vi "Selection Handle Mouse Down.vi"(7 "Shift?":bool, 8 "error in (no error)":errorcluster, 9 "Mouse Button":u16, 10 "Mouse Coords":T1, 11 "Listbox or Tree":refnum<vi>) -> (0 "error out":errorcluster, 3 "Discard?":bool)   [LabVIEW 2020, in "UI_ItemSelect.lvlib"]
uses:
  UI_ItemSelect.lvlib
  <vilib>/Utility/miscctls.llb/LVPoint32TypeDef.ctl
  SubVIs/item select mouse down data.ctl
  SubVIs/item select action.ctl
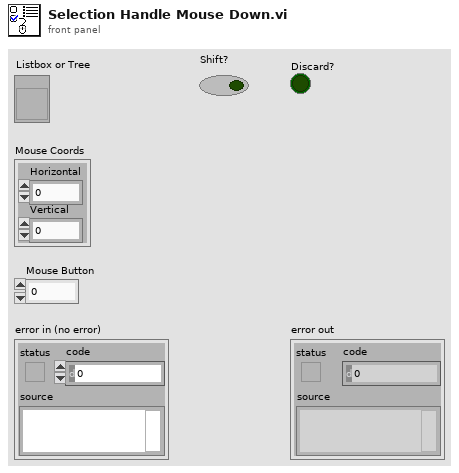
[diagram p1: front panel]
types:
  T1 = typedef "LVPoint32TypeDef.ctl" = cluster{"Horizontal":i32, "Vertical":i32}
  T2 = typedef "UI_ItemSelect.lvlib/item select action.ctl" = enum16{"init", "read", "write states", "write locks", "mouse down", "delete", "select all", "select none", "invert selection"}
  T3 = typedef "UI_ItemSelect.lvlib/item select mouse down data.ctl" = cluster{"Shift":bool, "Selected Row":i32}
  T4 = typedef "LVRowAndColumnTypeDef.ctl" = cluster{"Row":i32, "Column":i32}
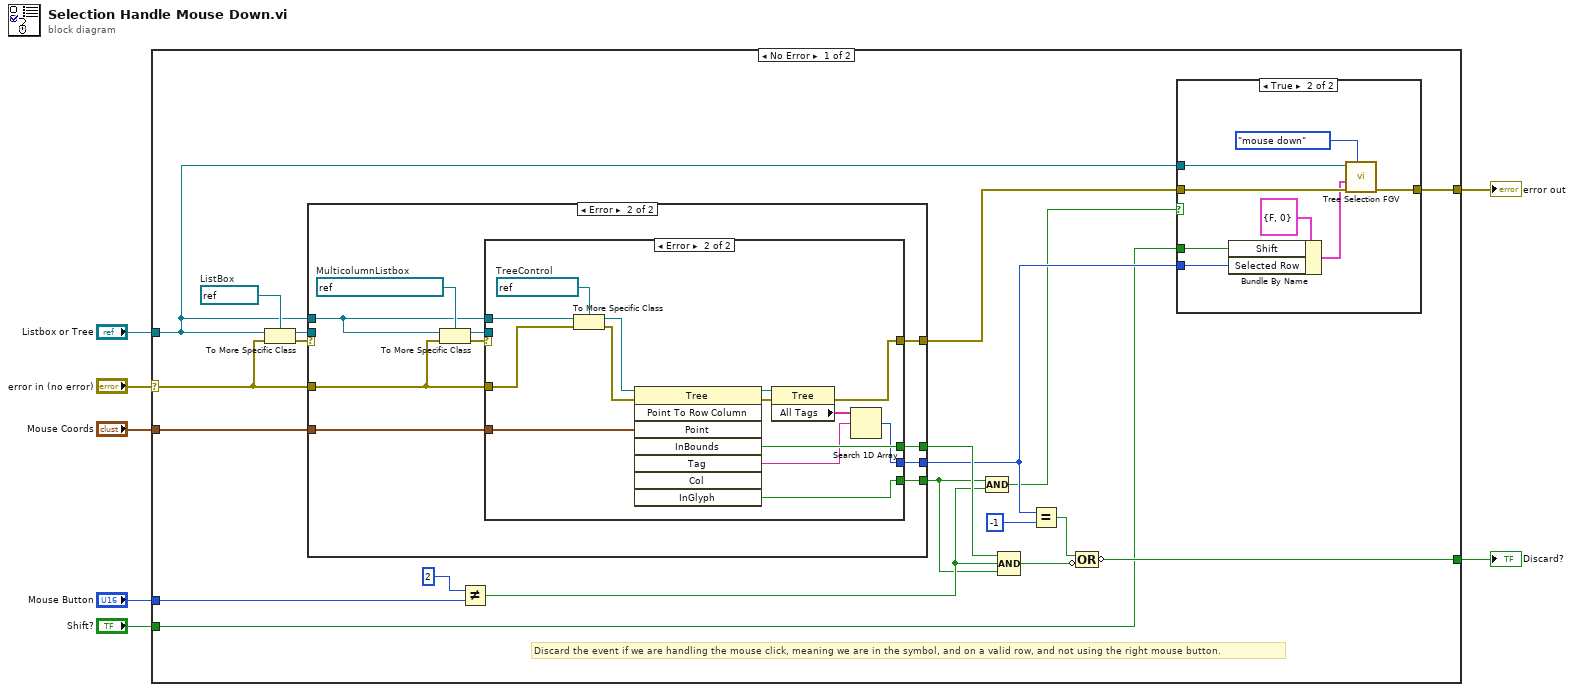
[diagram p0: block diagram]
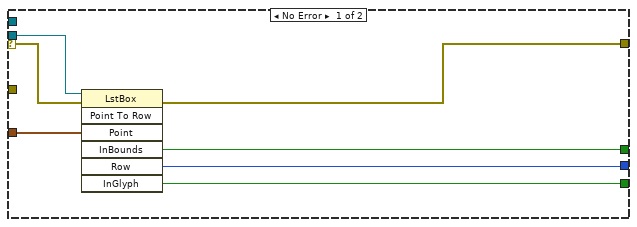
[diagram p2: hidden frame]
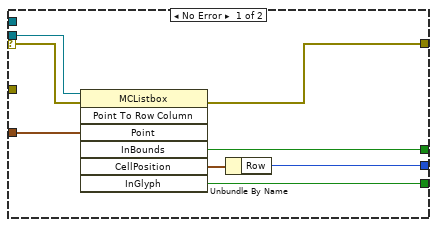
[diagram p3: hidden frame]
diagram:
  n1 = case shown="No Error" "error in (no error)" {
    selector: "error in (no error)" -> [w24 w76]
    tunnel: [w12 w76] -> w7
    tunnel: "Listbox or Tree" -> [w9 _]
    tunnel: "Mouse Coords" -> [w23 _]
    tunnel: "Mouse Button" -> [w22 _]
    tunnel: [w11 _] -> w2
    tunnel: "Shift?" -> [w10 _]
    frame No Error {
      w25 = refnum<vi> refnum  # ListBox
      # "Discard the event if we are handling the mouse click, meaning we are in the symbol, and on a valid row, and not using the right mouse button."
      n2 = To More Specific Class(target class=w25, reference=w9, error in=w24) -> (specific class reference=w27:refnum<vi>, error out=w26:errorcluster)
      n3 = case shown="Error" w26 {
        selector: w26 -> [w33 _]
        tunnel: w27 -> [w34 _]
        tunnel: w24 -> [_ w35]
        tunnel: [w32 w42] -> w15
        tunnel: w23 -> [w31 w41]
        tunnel: [w30 w39] -> w8
        tunnel: [w29 w40] -> w14
        tunnel: [w28 w38] -> w20
        tunnel: w9 -> [_ w36]
        frame No Error {
          n4 = invoke class="LstBox" method="Point To Row"(reference=w34, error in=w33, "Point"=w31) -> (error out=w32:errorcluster, "InBounds"=w28:bool, "Row"=w29:i32, "InGlyph"=w30:bool)  [unwired: 4 in, 3 out]
        }
        frame Error {
          w44 = refnum<vi> refnum  # MulticolumnListbox
          n5 = To More Specific Class(target class=w44, reference=w36, error in=w35) -> (specific class reference=w43:refnum<vi>, error out=w37:errorcluster)
          n6 = case shown="Error" w37 {
            selector: w37 -> [w45 _]
            tunnel: w43 -> [w52 _]
            tunnel: [w51 w53] -> w42
            tunnel: w41 -> [w50 w62]
            tunnel: [w48 w58] -> w40
            tunnel: [w47 w60] -> w39
            tunnel: [w46 w61] -> w38
            tunnel: w36 -> [_ w65]
            tunnel: w35 -> [_ w64]
            frame No Error {
              n7 = invoke class="MCListbox" method="Point To Row Column"(reference=w52, error in=w45, "Point"=w50) -> (error out=w51:errorcluster, "InBounds"=w46:bool, "CellPosition"=w49:T4, "InGlyph"=w47:bool)  [unwired: 4 in, 3 out]
              n8 = Unbundle By Name(w49) -> ("Row"=w48:i32)
            }
            frame Error {
              w66 = refnum<vi> refnum  # TreeControl
              n9 = To More Specific Class(target class=w66, reference=w65, error in=w64) -> (specific class reference=w57:refnum<vi>, error out=w63:errorcluster)
              n10 = invoke class="Tree" method="Point To Row Column"(reference=w57, error in=w63, "Point"=w62) -> (reference out=w56:refnum<vi>, error out=w55:errorcluster, "InBounds"=w61:bool, "Tag"=w59:string, "InGlyph"=w60:bool)  [unwired: 5 in, 3 out]
              n11 = property class="Tree"(reference=w56, error in=w55) -> (error out=w53:errorcluster, "All Tags"=w54:string[])  [unwired: 1 out]
              n12 = Search 1D Array(1D array=w54, element=w59) -> (index of element=w58:i32)  [unwired: 1 in]
            }
          }
        }
      }
      n13 = Not Equal?(x=u16 2, y=w22) -> (x != y?=w16:bool)
      n14 = Compound Arithmetic op=AND(w8, w16) -> (w13:bool)
      n15 = Compound Arithmetic op=AND(w20, w16, w8) -> (w19:bool)
      n16 = Equal?(x=w14, y=-1) -> (x = y?=w17:bool)
      n17 = Compound Arithmetic op=OR(w17, invert w19) -> (invert w11:bool)
      n18 = case shown="True" w13 {
        tunnel: w15 -> [w67 w70]
        tunnel: w9 -> [_ w73]
        tunnel: w14 -> [_ w71]
        tunnel: [w67 w69] -> w12
        tunnel: w10 -> [_ w72]
        frame False {
        }
        frame True {
          n19 = Bundle By Name(cluster=T3 {"Shift"=FALSE, "Selected Row"=0} ("Mouse down data"), "Shift"=w72, "Selected Row"=w71) -> (w68:T3)
          n20 = call "Tree Selection FGV.vi"("Action"=item_select_action."mouse down", "error in (no error)"=w70, "Mouse down data"=w68, "Listbox or Tree"=w73) -> ("error out"=w69:errorcluster)  [unwired: 6 in, 1 out]
        }
      }
    }
    frame Error {
    }
  }
  "error out" <- w7
  "Discard?" <- w2
